vi "JSON to LVObject - Dictionary of Object hierarchy - Returns Object.vi"() -> ()   [LabVIEW 2017, in "Generic Object Serializer Tests.lvlib" / "Type Name Handling.lvlib"]
uses:
  Generic Object Serializer/Generic Object Serializer.lvclass
  Dictionary/Dictionary.lvclass
  Generic Object Serializer/Type Name Handling.ctl
  Generic Object Serializer/Generic Object Serializer.lvclass/Generic Object Serializer.ctl
  Generic Object Serializer/Write Type Name Handling.vi
  Temperature Forecast/Temperature Forecast.lvclass
  C:/Users/de200256/Code/logmanoriginal/jsontext-object-serialization/Generic Object Serializer Tests/Weather Forecast/Weather Forecast.lvclass
  <vilib>/addons/_JKI Toolkits/Caraya/classes/Assert/Assert Equal Value and Type_Variant.vi
  Type Name Handling/Type Name Handling.lvlib
  <vilib>/addons/_JKI Toolkits/Caraya/classes/Test/Test.lvclass
  <vilib>/addons/_JKI Toolkits/Caraya/classes/Assert/Assert.lvclass
  Country/Country.lvclass
  City/City.lvclass
  Weather Forecast/Weather Forecast.lvclass
panel:
  out "error out":errorcluster
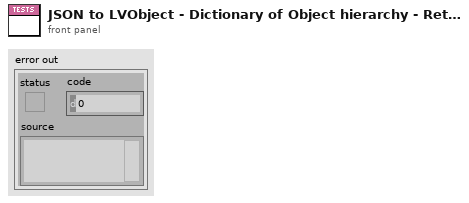
[diagram p1: front panel]
types:
  T1 = typedef "Generic Object Serializer.lvclass/Type Name Handling.ctl" = enum16{"None", "Inline"}
  T2 = cluster{string, "Country":refnum<class "Country.lvclass">}
  T3 = cluster{string, "LabVIEW Object":refnum<class>}[]
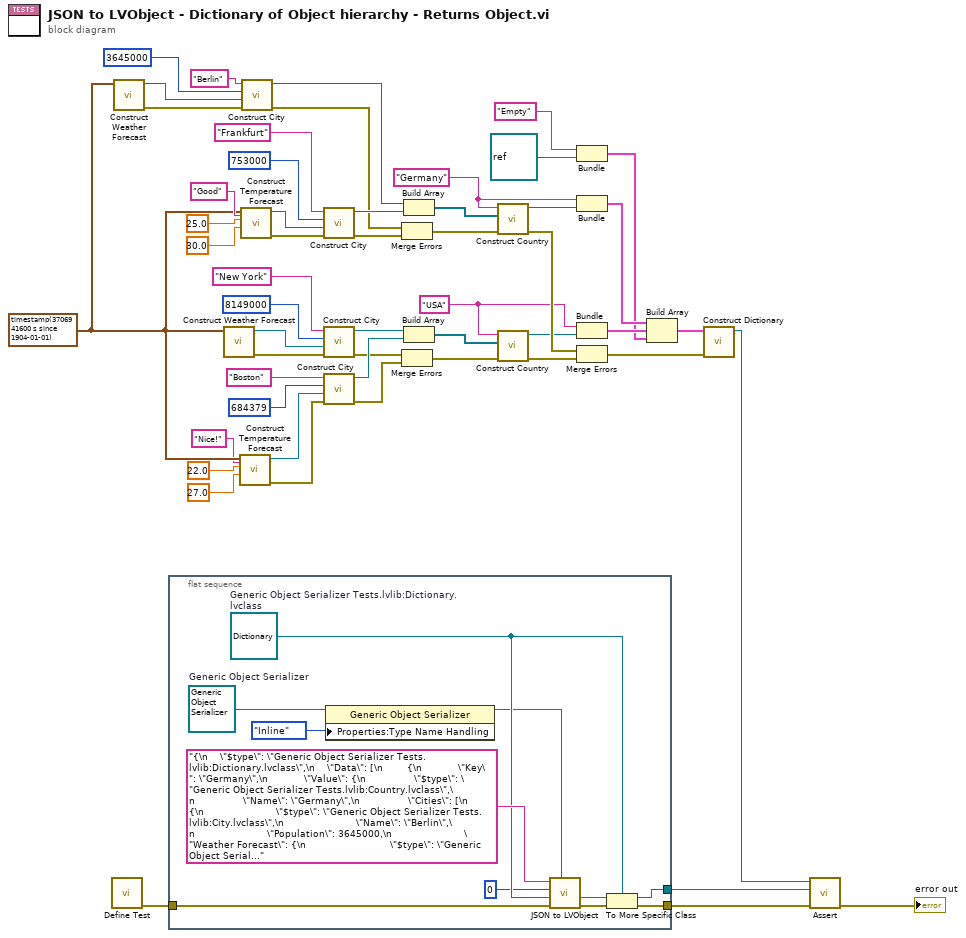
[diagram p0: block diagram]
diagram:
  w24 = "USA"
  w12 = timestamp(3706941600 s since 1904-01-01) ("Date")
  w47 = "Germany"
  n1 = call <vilib>:"Define Test.vi"() -> ("error out"=w53:errorcluster)  [unwired: 11 in]
  n2 = call "Construct Weather Forecast.vi"("Date"=w12) -> ("error out"=w34:errorcluster, "Weather Forecast"=w33:refnum<class "Weather Forecast.lvclass">)  [unwired: 9 in]
  n3 = flat-sequence {
    tunnel: w53 -> [w58]
    tunnel: [w57] -> w51
    tunnel: [w56] -> w50
    frame #0 {
      w61 = refnum<class "Dictionary.lvclass"> refnum  # Generic Object Serializer Tests.lvlib:Dictionary.lvclass
      w59 = refnum<class "Generic Object Serializer.lvclass"> refnum  # Generic Object Serializer
      n4 = property class="Generic Object Serializer"(reference=w59, "Properties:Type Name Handling"=Type_Name_Handling."Inline" ("Type Name Handling")) -> (reference out=w55:refnum<class "Generic Object Serializer.lvclass">)  [unwired: 1 in, 1 out]
      n5 = call-dynamic "JSON to LVObject.vi"("LVClass Serializer"=w55, "error in (no error)"=w58, "Object Type"=w61, "Offset"=0, "JSON"="{\n    \"$type\": \"Generic Object Serializer Tests.lvlib:Dictionary.lvclass\",\n    \"Data\": [\n        {\n            \"Key\": \"Germany\",\n            \"Value\": {\n                \"$type\": \"Generic Object Serializer Tests.lvlib:Country.lvclass\",\n                \"Name\": \"Germany\",\n                \"Cities\": [\n                    {\n                        \"$type\": \"Generic Object Serializer Tests.lvlib:City.lvclass\",\n                        \"Name\": \"Berlin\",\n                        \"Population\": 3645000,\n                        \"Weather Forecast\": {\n                            \"$type\": \"Generic Object Serializer Tests.lvlib:Weather Forecast.lvclass\",\n                            \"Date\": \"2021-06-19T10:00:00.000Z\"\n                        }\n                    },\n                    {\n                        \"$type\": \"Generic Object Serializer Tests.lvlib:City.lvclass\",\n                        \"Name\": \"Frankfurt\",\n                        \"Population\": 753000,\n                        \"Weather Forecast\": {\n                            \"$type\": \"Generic Object Serializer Tests.lvlib:Temperature Forecast.lvclass\",\n                            \"Date\": \"2021-06-19T10:00:00.000Z\",\n                            \"Temperature\": 25,\n                            \"Feels Like\": 30,\n                            \"Description\": \"Good\"\n                        }\n                    }\n                ]\n            }\n        },\n        {\n            \"Key\": \"USA\",\n            \"Value\": {\n                \"$type\": \"Generic Object Serializer Tests.lvlib:Country.lvclass\",\n                \"Name\": \"USA\",\n                \"Cities\": [\n                    {\n                        \"$type\": \"Generic Object Serializer Tests.lvlib:City.lvclass\",\n                        \"Name\": \"New York\",\n                        \"Population\": 8149000,\n                        \"Weather Forecast\": {\n                            \"$type\": \"Generic Object Serializer Tests.lvlib:Weather Forecast.lvclass\",\n                            \"Date\": \"2021-06-19T10:00:00.000Z\"\n                        }\n                    },\n                    {\n                        \"$type\": \"Generic Object Serializer Tests.lvlib:City.lvclass\",\n                        \"Name\": \"Boston\",\n                        \"Population\": 684379,\n                        \"Weather Forecast\": {\n                            \"$type\": \"Generic Object Serializer Tests.lvlib:Temperature Forecast.lvclass\",\n                            \"Date\": \"2021-06-19T10:00:00.000Z\",\n                            \"Temperature\": 22,\n                            \"Feels Like\": 27,\n                            \"Description\": \"Nice!\"\n                        }\n                    }\n                ]\n            }\n        },\n        {\n            \"Key\": \"Empty\",\n            \"Value\": {\n                \"$type\": \"LabVIEW Object\"\n            }\n        }\n    ]\n}") -> ("error out"=w64:errorcluster, "Object"=w62:refnum<class>)  [unwired: 5 in]
      n6 = To More Specific Class(target class=w61, reference=w62, error in=w64) -> (specific class reference=w56:refnum<class "Dictionary.lvclass">, error out=w57:errorcluster)
    }
  }
  n7 = call "Construct Weather Forecast.vi"("Date"=w12) -> ("error out"=w5:errorcluster, "Weather Forecast"=w14:refnum<class "Weather Forecast.lvclass">)  [unwired: 9 in]
  n8 = call "Construct Temperature Forecast.vi"("Description"="Nice!", "Feels Like [°C]"=27.0, "Temperature [°C]"=22.0, "Date"=w12) -> ("error out"=w4:errorcluster, "Temperature Forecast"=w13:refnum<class "Temperature Forecast.lvclass">)  [unwired: 6 in]
  n9 = call "Construct Temperature Forecast.vi"("Description"="Good", "Feels Like [°C]"=30.0, "Temperature [°C]"=25.0, "Date"=w12) -> ("error out"=w29:errorcluster, "Temperature Forecast"=w30:refnum<class "Temperature Forecast.lvclass">)  [unwired: 6 in]
  n10 = call "Construct City.vi"("error in (no error)"=w34, "Weather Forecast"=w33, "Population"=u32 3645000, "Name"="Berlin") -> ("error out"=w44:errorcluster, "City"=w46:refnum<class "City.lvclass">)  [unwired: 6 in]
  n11 = call "Construct City.vi"("error in (no error)"=w29, "Weather Forecast"=w30, "Population"=u32 753000, "Name"="Frankfurt") -> ("error out"=w43:errorcluster, "City"=w45:refnum<class "City.lvclass">)  [unwired: 6 in]
  n12 = call "Construct City.vi"("error in (no error)"=w5, "Weather Forecast"=w14, "Population"=u32 8149000, "Name"="New York") -> ("error out"=w8:errorcluster, "City"=w20:refnum<class "City.lvclass">)  [unwired: 6 in]
  n13 = call "Construct City.vi"("error in (no error)"=w4, "Weather Forecast"=w13, "Population"=u32 684379, "Name"="Boston") -> ("error out"=w7:errorcluster, "City"=w19:refnum<class "City.lvclass">)  [unwired: 6 in]
  n14 = Merge Errors(w44, w43) -> (w42:errorcluster)
  n15 = Merge Errors(w8, w7) -> (w6:errorcluster)
  n16 = Build Array(w46, w45) -> (w41:refnum<class "City.lvclass">[])
  n17 = Build Array(w20, w19) -> (w21:refnum<class "City.lvclass">[])
  n18 = call "Construct Country.vi"("error in (no error)"=w42, "Cities"=w41, "Name"=w47) -> ("error out"=w38:errorcluster, "Country"=w48:refnum<class "Country.lvclass">)  [unwired: 7 in]
  n19 = call "Construct Country.vi"("error in (no error)"=w6, "Cities"=w21, "Name"=w24) -> ("error out"=w22:errorcluster, "Country"=w25:refnum<class "Country.lvclass">)  [unwired: 7 in]
  n20 = Bundle("Empty", "LabVIEW Object"=refnum<class> refnum) -> (w1:cluster{string, "LabVIEW Object":refnum<class>})  [unwired: 1 in]
  n21 = Bundle(w47, "Country"=w48) -> (w40:T2)  [unwired: 1 in]
  n22 = Bundle(w24, "Country"=w25) -> (w23:T2)  [unwired: 1 in]
  n23 = Merge Errors(w38, w22) -> (w37:errorcluster)
  n24 = Build Array(w40, w23, w1) -> (w39:T3)
  n25 = call "Construct Dictionary.vi"("error in (no error)"=w37, "Data"=w39) -> ("Dictionary"=w49:refnum<class "Dictionary.lvclass">)  [unwired: 8 in, 1 out]
  n26 = call-poly <vilib>:"Assert.vi"("error in (no error)"=w51, "Y"=w50, "X"=w49) -> ("error out"=→"error out":errorcluster)  [unwired: 8 in]
